vi "Read_SaveDataPath.vi"(8 "error in (no error)":errorcluster caption="错误输入（无错误）") -> (0 "error out":errorcluster caption="错误输出", 3 "路径":path)   [LabVIEW 2018]
uses:
  Global.vi
  <vilib>/Utility/config.llb/Read Key (String).vi
  <vilib>/Utility/config.llb/NI_LVConfig.lvlib
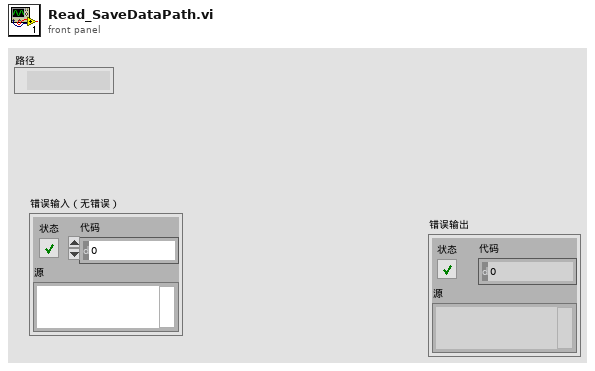
[diagram p1: front panel]
types:
  T1 = typedef "NI_LVConfig.lvlib/Config Data RefNum.ctl" = refnum<k1>
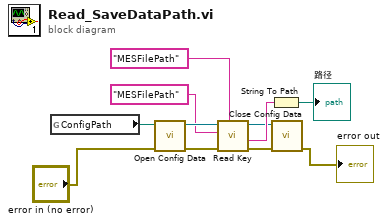
[diagram p0: block diagram]
diagram:
  n1 = global read "Global.vi" "ConfigPath"() -> (w9:path)
  n2 = call <vilib>:"Open Config Data.vi"("error in (no error)"="error in (no error)", "configuration file path"=w9) -> ("error out"=w3:errorcluster, "refnum"=w7:T1)  [unwired: 7 in, 1 out]
  n3 = call-poly <vilib>:"Read Key.vi"("section"="MESFilePath", "error in (no error)"=w3, "key"="MESFilePath", "refnum"=w7) -> ("error out"=w4:errorcluster, "value"=w10:string, "refnum out"=w8:T1)  [unwired: 4 in, 1 out]
  n4 = String To Path(string=w10) -> (path=→"路径":path)
  n5 = call <vilib>:"Close Config Data.vi"("error in (no error)"=w4, "refnum"=w8) -> ("error out"=→"error out":errorcluster)  [unwired: 8 in, 1 out]
